vi "Get Array Size.vi"(8 "error in (no error)":errorcluster, 11 "JSON Array in":refnum<class "JSON Array.lvclass">) -> (0 "error out":errorcluster, 2 "size(s)":i32, 3 "JSON Array out":refnum<class "JSON Array.lvclass">)   [LabVIEW 2017, in "LVJSON.lvlib" / "JSON Array.lvclass"]
uses:
  JSON Array.lvclass
  JSON Array.lvclass/JSON Array.ctl
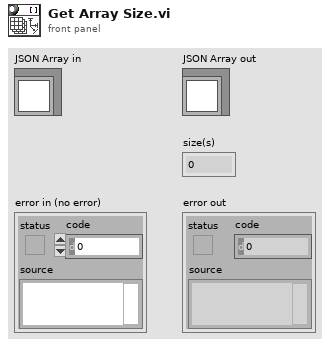
[diagram p1: front panel]
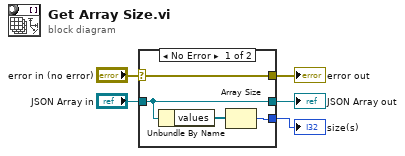
[diagram p0: block diagram]
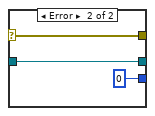
[diagram p2: hidden frame]
diagram:
  n1 = case shown="No Error" "error in (no error)" {
    selector: "error in (no error)" -> [w9 w12]
    tunnel: [w9 w12] -> w4
    tunnel: [w8 w11] -> w2
    tunnel: "JSON Array in" -> [w8 w11]
    tunnel: [w6 0] -> w1
    frame No Error {
      n2 = Unbundle By Name(w8) -> ("values"=w7:refnum<class "JSON Datatype.lvclass">[])
      n3 = Array Size(array=w7) -> (size(s)=w6:i32)
    }
    frame Error {
    }
  }
  "error out" <- w4
  "JSON Array out" <- w2
  "size(s)" <- w1
